vi "Read and Display Unicode Files.vi"() -> ()   [LabVIEW 2017]
uses:
  <vilib>/Utility/miscctls.llb/LVPointTypeDef.ctl
panel:
  in  "Language File Path":path
  in  "Language Selection":T1(ring)=enum."Chinese (Simlified)"
  in  "Numeric":dbl caption="W[U^Nåe"
  in  "stop":bool
  out "Array of Strings with Force Unicode On":string[](array[string])
  out "Normal Array of Strings":string[](array[string])
  out "Raw String Read from File":string
  out "String with Force Unicode On":string
  out "Normal String":string
  # "Instruction:\n1. Select the path of Caption.txt (contains different languages to be explored)\n\n2. Run the VI\n\n3. Change the Language Selection List and observe the change of the indicators/captions"
  # "Observation:\nSet 1: This numeric indicator's caption changes according to the Language Selection.\n           This is done by setting its property's  \"Caption.InterpAsunicode\" to true on the block diagram\n\nSet 2: Caption.txt text is broken up into array elements. The second array display text in its original language\n           This is done by right clicking on the array and select \"Force Unicode Text\"\n\nSet 3: These 3 string indicators display Caption.txt directly. The first 2 indicators doesn't have \"Froce Unicode Text\"\n           Enabled and the 3rd one has it enabled by right clicking"
  # "Set 1:"
  # "Set 2:"
  # "Set 3:"
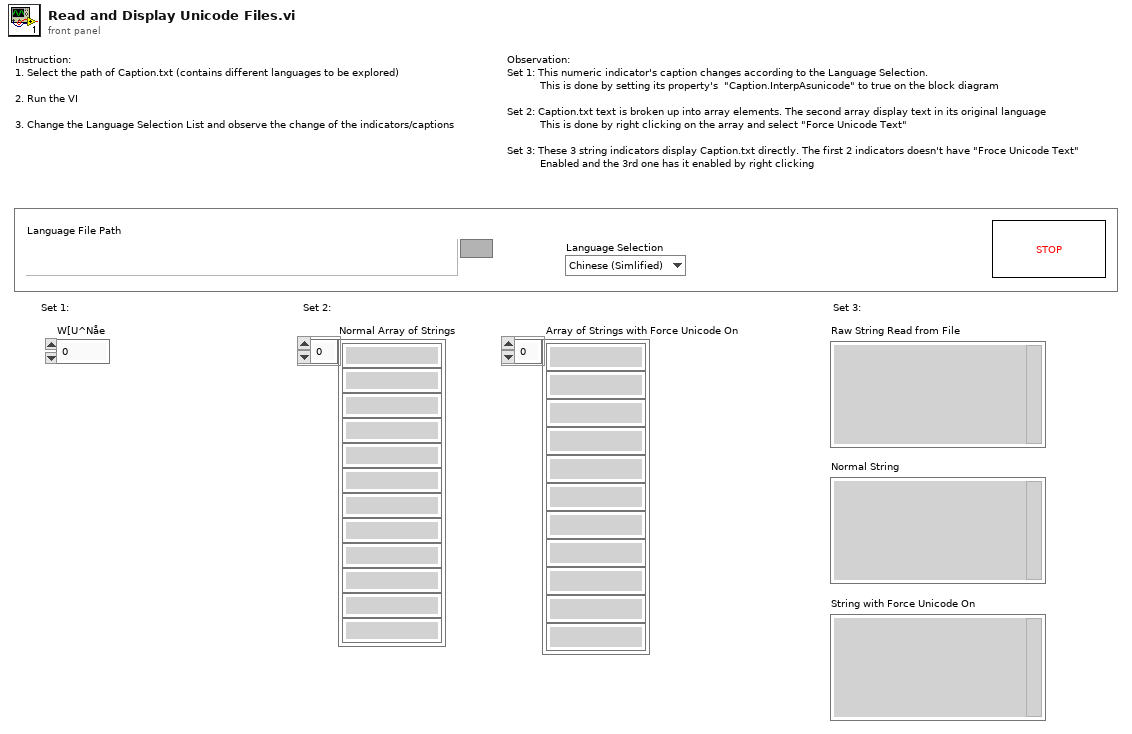
[diagram p1: front panel]
types:
  T1 = enum16{"English", "Russian", "Japanese", "Korean", "Chinese (Simlified)"}
  T2 = typedef "LVPointTypeDef.ctl" = cluster{"Horizontal":i16, "Vertical":i16}
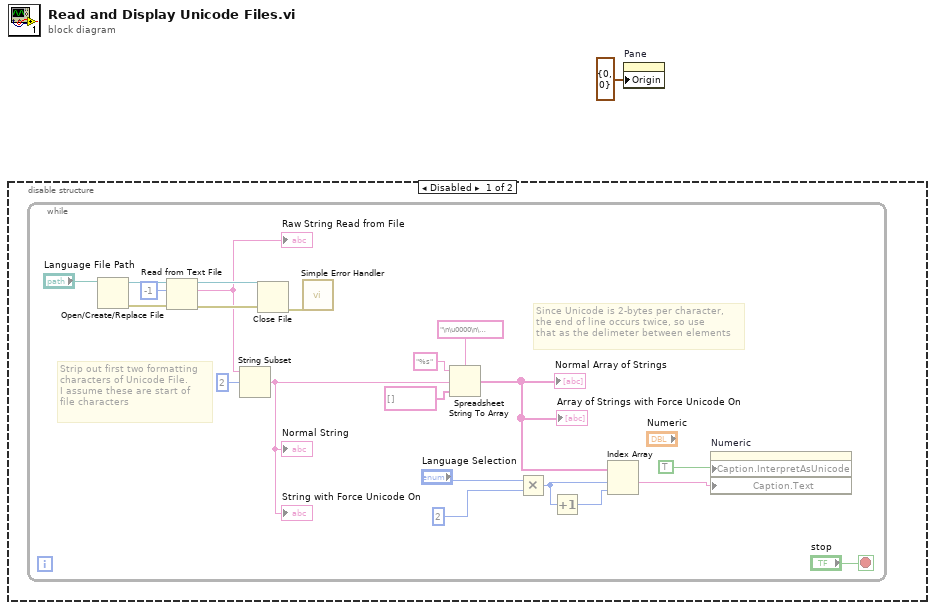
[diagram p0: block diagram]
diagram:
  n1 = disable-structure shown="Disabled" {
    frame Disabled {
      n2 = while {
        stop <- "stop" stop-if-true
        # "Since Unicode is 2-bytes per character,\nthe end of line occurs twice, so use\nthat as the delimeter between elements"
        # "Strip out first two formatting\ncharacters of Unicode File.\nI assume these are start of \nfile characters"
        n3 = Open/Create/Replace File(file path (use dialog)="Language File Path") -> (refnum out=w22:refnum<file>, error out=w19:errorcluster)  [unwired: 5 in, 1 out]
        n4 = Read from Text File(file (use dialog)=w22, count=-1, error in=w19) -> (refnum out=w20:refnum<file>, text=w15:string, error out=w18:errorcluster)  [unwired: 1 in, 1 out]
        "Raw String Read from File" <- w15
        n5 = String Subset(string=w15, offset (0)=2) -> (substring=w6:string)  [unwired: 1 in]
        "Normal String" <- w6
        "String with Force Unicode On" <- w6
        n6 = Close File(refnum=w20, error in=w18) -> (error out=w7:errorcluster)  [unwired: 1 out]
        n7 = call <vilib>:"Simple Error Handler.vi"("error in (no error)"=w7) -> ()  [unwired: 4 in, 5 out]
        n8 = Spreadsheet String To Array(delimiter (Tab)="\n\u0000\n\u0000", format string="%s", spreadsheet string=w6, array type (2D Dbl)=string[] []) -> (array=w8:string[])
        "Normal Array of Strings" <- w8
        "Array of Strings with Force Unicode On" <- w8
        n9 = Multiply(x="Language Selection", y=2) -> (x*y=w11:i32)
        n10 = Increment(x=w11) -> (x+1=w10:i32)
        n11 = Index Array(array=w8, index #1=w11, index #2=w10) -> (element #1=w3:string)  [unwired: 1 out]
        n12 = property on="Numeric" class="DigNum (strict)"("Caption.InterpretAsUnicode"=TRUE ("Numeric 1: Caption.Interpret As Unicode?"), "Caption.Text"=w3) -> ()  [unwired: 2 in, 2 out]
      }
    }
    frame Enabled {
    }
  }
  n13 = property on="Pane" class="Pane"("Origin"=T2 {"Horizontal"=0, "Vertical"=0}) -> ()  [unwired: 2 in, 2 out]
